vi "Comp_Group_Motion.vi"(5 "stop 2":refnum<vi>, 6 "Slave Axis":i32, 7 "Master Axis":i32, 8 "error in (no error)":errorcluster, 9 "Motionphase":T1(array[cluster]), 10 "Group Cluster":T2, 11 "VISA resource name in":refnum<visa-resource-name>) -> (0 "error out":errorcluster, 3 "VISA resource name out":refnum<visa-resource-name>)   [LabVIEW 2011]
uses:
  <instrlib>/Newport ESP301/Newport ESP301.lvlib
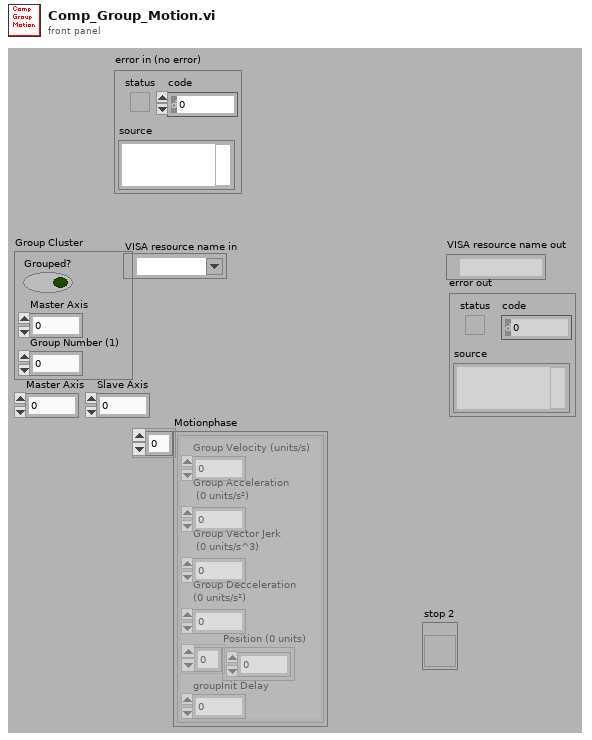
[diagram p1: front panel]
types:
  T1 = cluster{"Group Velocity (units/s)":dbl, "Group Acceleration\n (0 units/s²) ":dbl, "Group Vector Jerk\n (0 units/s^3)":dbl, "Group Decceleration \n(0 units/s²)":dbl, "Position (0 units)":dbl[], "groupInit Delay":u32}[]
  T2 = cluster{"Grouped?":bool, "Master Axis":i32, "Group Number (1)":i32}
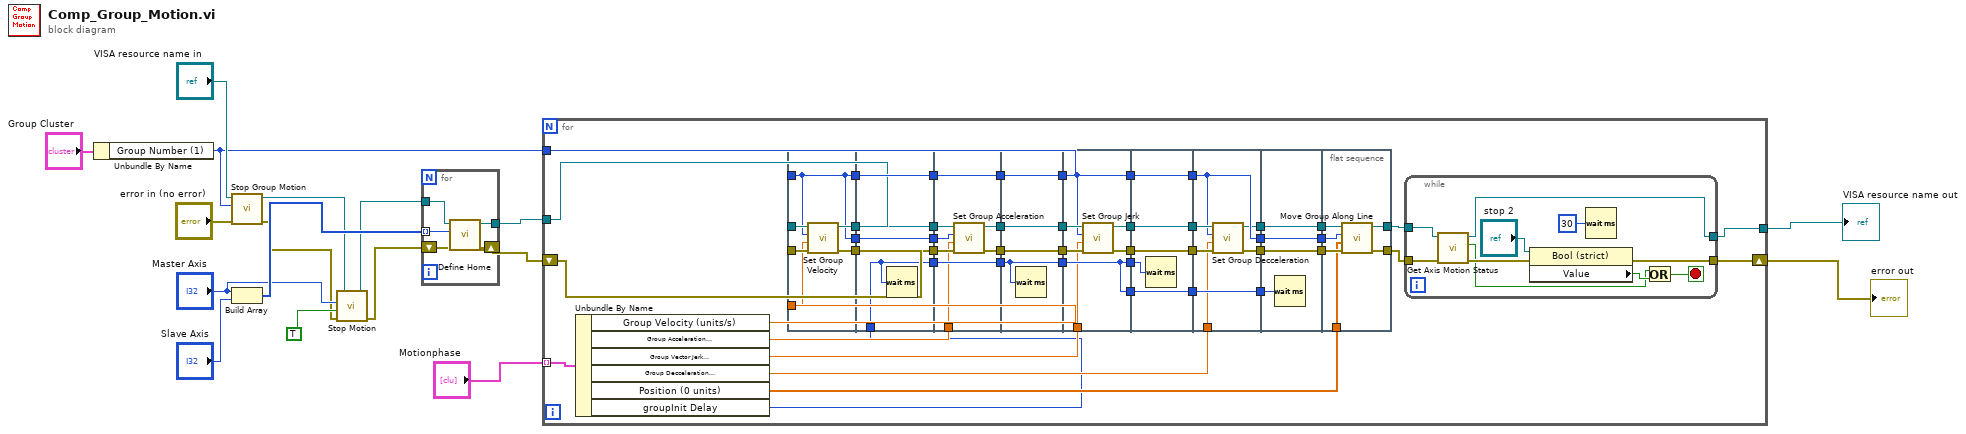
[diagram p0: block diagram]
diagram:
  n1 = Unbundle By Name("Group Cluster") -> ("Group Number (1)"=w12:i32)
  n2 = call <instrlib>:"Stop Group Motion.vi"("error in (no error)"="error in (no error)", "Group Number (1)"=w12, "VISA resource name"="VISA resource name in") -> ("error out"=w6:errorcluster, "VISA resource name out"=w4:refnum<visa-resource-name>)  [unwired: 3 in]
  n3 = Build Array("Master Axis", "Slave Axis") -> (w14:i32[])
  n4 = call <instrlib>:"Stop Motion.vi"("error in (no error)"=w6, "Stop all axes (F)"=TRUE, "Axis (1)"="Master Axis", "VISA resource name"=w4) -> ("error out"=w5:errorcluster, "VISA resource name out"=w3:refnum<visa-resource-name>)  [unwired: 2 in]
  n5 = for {
    tunnel: w14 -> [w22] mode=indexing
    tunnel: w3 -> [w21]
    tunnel: [w18] -> w11
    shift-right: [w19] -> w1
    shift-left: w5 -> [w20]
    n6 = call <instrlib>:"Define Home.vi"("error in (no error)"=w20, "Axis (1)"=w22, "VISA resource name"=w21) -> ("error out"=w19:errorcluster, "VISA resource name out"=w18:refnum<visa-resource-name>)  [unwired: 3 in]
  }
  n7 = for {
    tunnel: "Motionphase" -> [w36] mode=indexing
    tunnel: w12 -> [w29]
    tunnel: w11 -> [w28]
    tunnel: [w25] -> w10
    shift-right: [w24] -> w2
    shift-left: w1 -> [w23]
    n8 = Unbundle By Name(w36) -> ("Group Velocity (units/s)"=w35:dbl, "Group Acceleration\n (0 units/s²)"=w34:dbl, "Group Vector Jerk\n (0 units/s^3)"=w33:dbl, "Group Decceleration \n(0 units/s²)"=w32:dbl, "Position (0 units)"=w31:dbl[], "groupInit Delay"=w30:u32)
    n9 = flat-sequence {
      tunnel: w28 -> [w85]
      tunnel: w29 -> [w81]
      tunnel: w23 -> [w84]
      tunnel: [w83] -> w69
      tunnel: [w82] -> w68
      tunnel: [w81] -> w67
      tunnel: [w81] -> w66
      tunnel: w35 -> [w80]
      tunnel: w69 -> [w90]
      tunnel: [w90] -> w65
      tunnel: w68 -> [w89]
      tunnel: [w89] -> w64
      tunnel: w67 -> [w88]
      tunnel: [w88] -> w63
      tunnel: w66 -> [w87]
      tunnel: [w87] -> w62
      tunnel: [w86] -> w61
      tunnel: w30 -> [w86]
      tunnel: w65 -> [w98]
      tunnel: [w97] -> w60
      tunnel: w64 -> [w96]
      tunnel: [w95] -> w59
      tunnel: w63 -> [w94]
      tunnel: [w93] -> w58
      tunnel: w62 -> [w93]
      tunnel: w61 -> [w92]
      tunnel: [w92] -> w57
      tunnel: w34 -> [w91]
      tunnel: w60 -> [w102]
      tunnel: [w102] -> w56
      tunnel: w59 -> [w101]
      tunnel: [w101] -> w55
      tunnel: w58 -> [w100]
      tunnel: [w100] -> w54
      tunnel: w57 -> [w99]
      tunnel: [w99] -> w53
      tunnel: w56 -> [w109]
      tunnel: w55 -> [w108]
      tunnel: w54 -> [w106]
      tunnel: [w107] -> w52
      tunnel: [w106] -> w51
      tunnel: [w105] -> w50
      tunnel: [w104] -> w49
      tunnel: w53 -> [w104]
      tunnel: [w104] -> w48
      tunnel: w33 -> [w103]
      tunnel: [w114] -> w47
      tunnel: w52 -> [w114]
      tunnel: w51 -> [w113]
      tunnel: [w113] -> w46
      tunnel: w50 -> [w112]
      tunnel: [w112] -> w45
      tunnel: w49 -> [w111]
      tunnel: [w110] -> w44
      tunnel: w48 -> [w110]
      tunnel: w47 -> [w121]
      tunnel: w46 -> [w117]
      tunnel: w45 -> [w120]
      tunnel: [w119] -> w43
      tunnel: w44 -> [w119]
      tunnel: w32 -> [w118]
      tunnel: [w117] -> w42
      tunnel: [w116] -> w41
      tunnel: [w115] -> w40
      tunnel: w43 -> [w125]
      tunnel: [w124] -> w39
      tunnel: w42 -> [w124]
      tunnel: [w123] -> w38
      tunnel: w41 -> [w123]
      tunnel: [w122] -> w37
      tunnel: w40 -> [w122]
      tunnel: w39 -> [w131]
      tunnel: w38 -> [w130]
      tunnel: w37 -> [w129]
      tunnel: w31 -> [w128]
      tunnel: [w127] -> w27
      tunnel: [w126] -> w26
      frame #0 {
        n10 = call <instrlib>:"Set Group Velocity.vi"("error in (no error)"=w84, "Velocity (units/s)"=w80, "Group Number (1)"=w81, "VISA resource name"=w85) -> ("error out"=w82:errorcluster, "VISA resource name out"=w83:refnum<visa-resource-name>)  [unwired: 2 in]
      }
      frame #1 {
        n11 = Wait (ms)(milliseconds to wait=w86) -> ()  [unwired: 1 out]
      }
      frame #2 {
        n12 = call <instrlib>:"Set Group Acceleration.vi"("error in (no error)"=w96, "Acceleration (0 units/s²)"=w91, "Group Number (1)"=w94, "VISA resource name"=w98) -> ("error out"=w95:errorcluster, "VISA resource name out"=w97:refnum<visa-resource-name>)  [unwired: 2 in]
      }
      frame #3 {
        n13 = Wait (ms)(milliseconds to wait=w99) -> ()  [unwired: 1 out]
      }
      frame #4 {
        n14 = call <instrlib>:"Set Group Jerk.vi"("error in (no error)"=w108, "Vector Jerk (0 units/s^3)"=w103, "Group Number (1)"=w106, "VISA resource name"=w109) -> ("error out"=w105:errorcluster, "VISA resource name out"=w107:refnum<visa-resource-name>)  [unwired: 2 in]
      }
      frame #5 {
        n15 = Wait (ms)(milliseconds to wait=w111) -> ()  [unwired: 1 out]
      }
      frame #6 {
        n16 = call <instrlib>:"Set Group Decceleration.vi"("error in (no error)"=w120, "Decceleration (0 units/s²)"=w118, "Group Number (1)"=w117, "VISA resource name"=w121) -> ("error out"=w115:errorcluster, "VISA resource name out"=w116:refnum<visa-resource-name>)  [unwired: 2 in]
      }
      frame #7 {
        n17 = Wait (ms)(milliseconds to wait=w125) -> ()  [unwired: 1 out]
      }
      frame #8 {
        n18 = call <instrlib>:"Move Group Along Line.vi"("error in (no error)"=w129, "Position (0 units)"=w128, "Group Number (1)"=w131, "VISA resource name"=w130) -> ("error out"=w126:errorcluster, "VISA resource name out"=w127:refnum<visa-resource-name>)  [unwired: 2 in]
      }
    }
    n19 = while {
      tunnel: w27 -> [w79]
      tunnel: [w77] -> w25
      tunnel: w26 -> [w78]
      tunnel: [w74] -> w24
      stop <- w71 stop-if-true
      n20 = call <instrlib>:"Get Axis Motion Status.vi"("error in (no error)"=w78, "VISA resource name"=w79) -> ("error out"=w75:errorcluster, "Motion Done"=w72:bool, "VISA resource name out"=w77:refnum<visa-resource-name>)  [unwired: 3 in]
      n21 = property class="Bool (strict)"(reference="stop 2", error in=w75) -> (error out=w74:errorcluster, "Value"=w73:bool)  [unwired: 1 out]
      n22 = Wait (ms)(milliseconds to wait=u32 30) -> ()  [unwired: 1 out]
      n23 = Or(x=w72, y=w73) -> (x .or. y?=w71:bool)
    }
  }
  "VISA resource name out" <- w10
  "error out" <- w2
